vi "AK-LNI Antwortstring teilen.vi"(11 "Antwortstring":string) -> (3 "Empfangsdaten":string[](array[string]))   [LabVIEW 2020, in "Linearisierung v2.lvlib" / "Gasteiler.lvlib" / "AK Komm Gasteiler.lvlib"]
doc: "Trennt den Antwortstring, in dem jedes Argument mit einem Leerzeichen beginnt, in die einzelnen Argumente auf. Die Empfangsdaten enthalten in jedem Arrayelement ein Argument als String."
uses:
  AK Komm Gasteiler.lvlib
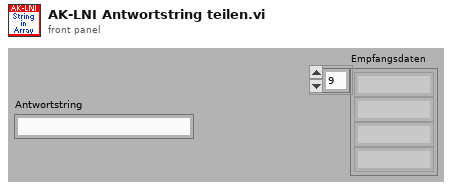
[diagram p1: front panel]
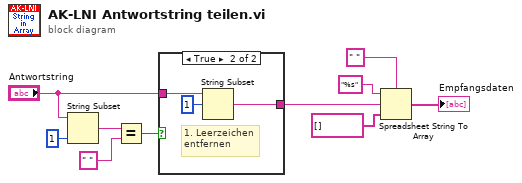
[diagram p0: block diagram]
diagram:
  n1 = String Subset(string="Antwortstring", length (rest)=1 ("Länge (Rest)")) -> (substring=w3:string)  [unwired: 1 in]
  n2 = Equal?(x=w3, y=" ") -> (x = y?=w1:bool)
  n3 = case shown="True" w1 {
    tunnel: "Antwortstring" -> [w11 w14]
    tunnel: [w11 w12] -> w7
    frame False {
    }
    frame True {
      # "1. Leerzeichen\nentfernen"
      n4 = String Subset(string=w14, offset (0)=1 ("Länge (Rest)")) -> (substring=w12:string)  [unwired: 1 in]
    }
  }
  n5 = Spreadsheet String To Array(delimiter (Tab)=" " ("Trennzeichen (Tabulator)"), format string="%s" ("Format-String"), spreadsheet string=w7, array type (2D Dbl)=string[] []) -> (array=→"Empfangsdaten":string[])
